vi "ATMonochromator_acceptCommand_calibrateWavelength.vi"(8 "error in (no error)":errorcluster, 11 "command_calibrateWavelength_Ctl":T1) -> (0 "error out":errorcluster, 2 "function return":i32, 3 "command_calibrateWavelength_Ctl out":T1)   [LabVIEW 2016, in "SALLV_ATMonochromator.lvlib"]
doc: "int ATMonochromator_shm_acceptCommand_calibrateWavelengthLV(ATMonochromator_command_calibrateWavelengthLV *command_calibrateWavelength_Ctl );"
uses:
  SALLV_ATMonochromator.lvlib
  DataTypes/command_calibrateWavelength.ctl
  SALLV_ATMonochromator.so
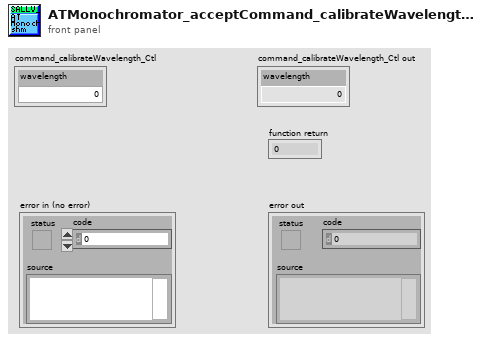
[diagram p1: front panel]
types:
  T1 = typedef "SALLV_ATMonochromator.lvlib/command_calibrateWavelength.ctl" = cluster{"wavelength":sgl}
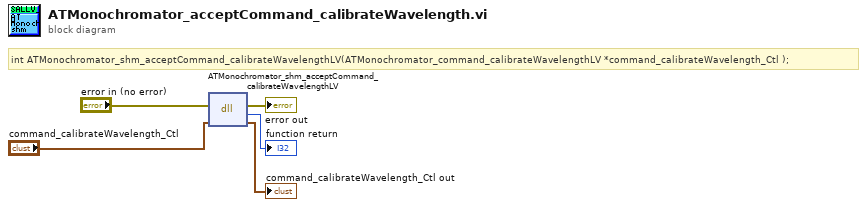
[diagram p0: block diagram]
diagram:
  # "int ATMonochromator_shm_acceptCommand_calibrateWavelengthLV(ATMonochromator_command_calibrateWavelengthLV *command_calibrateWavelength_Ctl );"
  n1 = dll-call lib="home/harini/tcs/SALLV_ATMonochromator/SALLV_ATMonochromator.*" fn="ATMonochromator_shm_acceptCommand_calibrateWavelengthLV"(error in="error in (no error)", "command_calibrateWavelength_Ctl"="command_calibrateWavelength_Ctl") -> (error out=→"error out":errorcluster, →"function return":i32, "command_calibrateWavelength_Ctl"=→"command_calibrateWavelength_Ctl out":T1)  [unwired: 2 in, 1 out]
